vi "User Event-Settings-Value Change.vi"(8 "Error In":errorcluster, 11 "Root Panel Actor in":refnum<class "Root Panel Actor.lvclass">) -> (0 "Error Out":errorcluster, 3 "Root Panel Actor out":refnum<class "Root Panel Actor.lvclass">)   [LabVIEW 2021, in "Root Panel.lvlib" / "Root Panel Actor.lvclass"]
uses:
  Root Panel Actor.lvclass
  C:/Program Files (x86)/National Instruments/LabVIEW 2021/vi.lib/MGI/Panel Manager/Panel Actor/Panel Actor/Panel Actor.lvclass
  C:/Users/Thomas/Documents/Projects/TemplateVIEW/Sources/Appearance Actor/Appearance Actor/Appearance Actor.lvclass
  Modules/Settings Module/Settings Actor/Settings Actor.lvclass
  Root Panel Actor.lvclass/Root Panel Actor.ctl
  Appearance Actor/Appearance Actor/Appearance Actor.lvclass/Appearance Actor.ctl
  Appearance Actor/Appearance Actor Messages/Recieve Theme From Caller Msg/Recieve Theme From Caller Msg.lvclass/Recieve Theme From Caller Msg.ctl
  <vilib>/ActorFramework/Message Enqueuer/Message Enqueuer.lvclass/Message Enqueuer.ctl
  <vilib>/ActorFramework/Message Enqueuer/Enqueue.vi
  <vilib>/MGI/Panel Manager/Panel/Panel/Subpanel/Subpanel.lvclass
  C:/Program Files (x86)/National Instruments/LabVIEW 2021/vi.lib/MGI/Panel Manager/Panel/Panel/Panel.lvclass
  Appearance Actor/Appearance Actor Messages/Recieve Theme From Caller Msg/Recieve Theme From Caller Msg.lvclass
  C:/Program Files (x86)/National Instruments/LabVIEW 2021/vi.lib/ActorFramework/Message/Message.lvclass
  <vilib>/MGI/Panel Manager/Panel/Panel/Subpanel/Subpanel.vi
  <vilib>/ActorFramework/Message Priority Queue/Priority Enqueue.vi
  Appearance Actor/Theme Classes/Generic Theme/Generic Theme.lvclass
  <vilib>/MGI/Panel Manager/Panel Actor/Panel Actor/Panel Actor.lvclass
  <vilib>/MGI/Panel Manager/Panel/Panel.lvlib
  Appearance Actor/Appearance Actor/Appearance Actor.lvclass
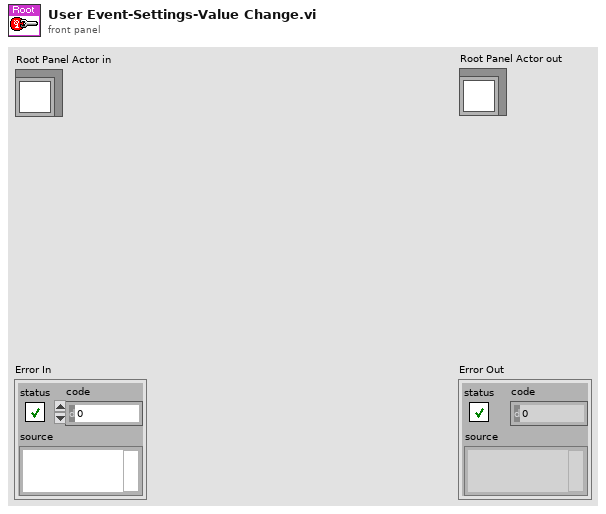
[diagram p1: front panel]
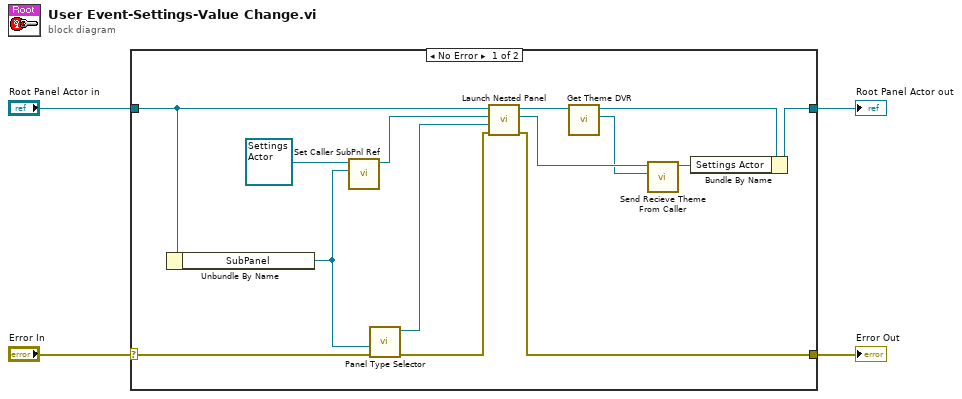
[diagram p0: block diagram]
diagram:
  n1 = case shown="No Error" "Error In" {
    selector: "Error In" -> [w16 w20]
    tunnel: [w17 w20] -> w1
    tunnel: [w18 w19] -> w3
    tunnel: "Root Panel Actor in" -> [w13 w19]
    frame No Error {
      n2 = Unbundle By Name(w13) -> ("SubPanel"=w5:refnum<vi>)
      n3 = call "Set Caller SubPnl Ref.vi"("Caller SubPnl Ref"=w5, "Appearance Actor in"=refnum<class "Settings Actor.lvclass"> refnum ("Settings Module.lvlib:Settings Actor.lvclass")) -> ("Appearance Actor out"=w6:refnum<class "Settings Actor.lvclass">)  [unwired: 8 in, 1 out]
      n4 = call-poly <vilib>:"Panel Type Selector.vi"("Error In"=w16, "Sub Panel"=w5) -> ("Error Out"=w15:errorcluster, "Subpanel Out"=w14:refnum<class "Subpanel.lvclass">)  [unwired: 8 in]
      n5 = call <vilib>:"Launch Nested Panel.vi"("error in (no error)"=w15, "Panel"=w14, "Nested Panel Actor"=w6, "Panel Actor in"=w13) -> ("error out"=w17:errorcluster, "Nested Actor's Enqueuer"=w12:refnum<class "Message Enqueuer.lvclass">, "Panel Actor out"=w10:refnum<class "Root Panel Actor.lvclass">)  [unwired: 4 in, 1 out]
      n6 = call "Get Theme DVR.vi"("Appearance Actor in"=w10) -> ("Theme DVR"=w8:refnum<data-value>, "Appearance Actor out"=w9:refnum<class "Root Panel Actor.lvclass">)  [unwired: 8 in, 1 out]
      n7 = call "Send Recieve Theme From Caller.vi"("Theme DVR"=w8, "Message Enqueuer"=w12) -> ("Message Enqueuer out"=w11:refnum<class "Message Enqueuer.lvclass">)  [unwired: 8 in, 1 out]
      n8 = Bundle By Name(cluster=w9, "Settings Actor"=w11) -> (w18:refnum<class "Root Panel Actor.lvclass">)
    }
    frame Error {
    }
  }
  "Error Out" <- w1
  "Root Panel Actor out" <- w3
